vi "test4-EndNodeHandlesErrorForNotAllowedMessages.vi"(8 "error in (no error)":errorcluster, 11 "TestCase in":refnum<class "testcase-CSMChainMode.lvclass">) -> (0 "error out":errorcluster, 3 "TestCase out":refnum<class "testcase-CSMChainMode.lvclass">)   [LabVIEW 2017, in "testcase-CSMChainMode.lvclass"]
uses:
  testcase-CSMChainMode.lvclass
  src/user.lib/_NEVSTOP/Communicable State Machine(CSM)/_Support/Typedef/_CSM_MODE.ctl
  8deca385-1376-47bb-b92d-c44567c1a462.vi
  <vilib>/addons/_JKI Toolkits/VI Tester/TestCase.llb/TestCase.lvclass
  src/user.lib/_NEVSTOP/Communicable State Machine(CSM)/Communicable State Machine.lvlib
  C:/Program Files (x86)/National Instruments/LabVIEW 2017/vi.lib/addons/_JKI Toolkits/VI Tester/TestCase.llb/TestCase.lvclass
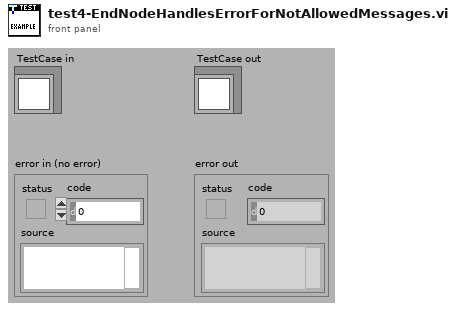
[diagram p1: front panel]
types:
  T1 = typedef "Communicable State Machine.lvlib/_CSM_MODE.ctl" = enum16{"Not Exist", "Stand Alone", "CSM", "Worker", "Worker Agent", "Chain Node", "Chain"}
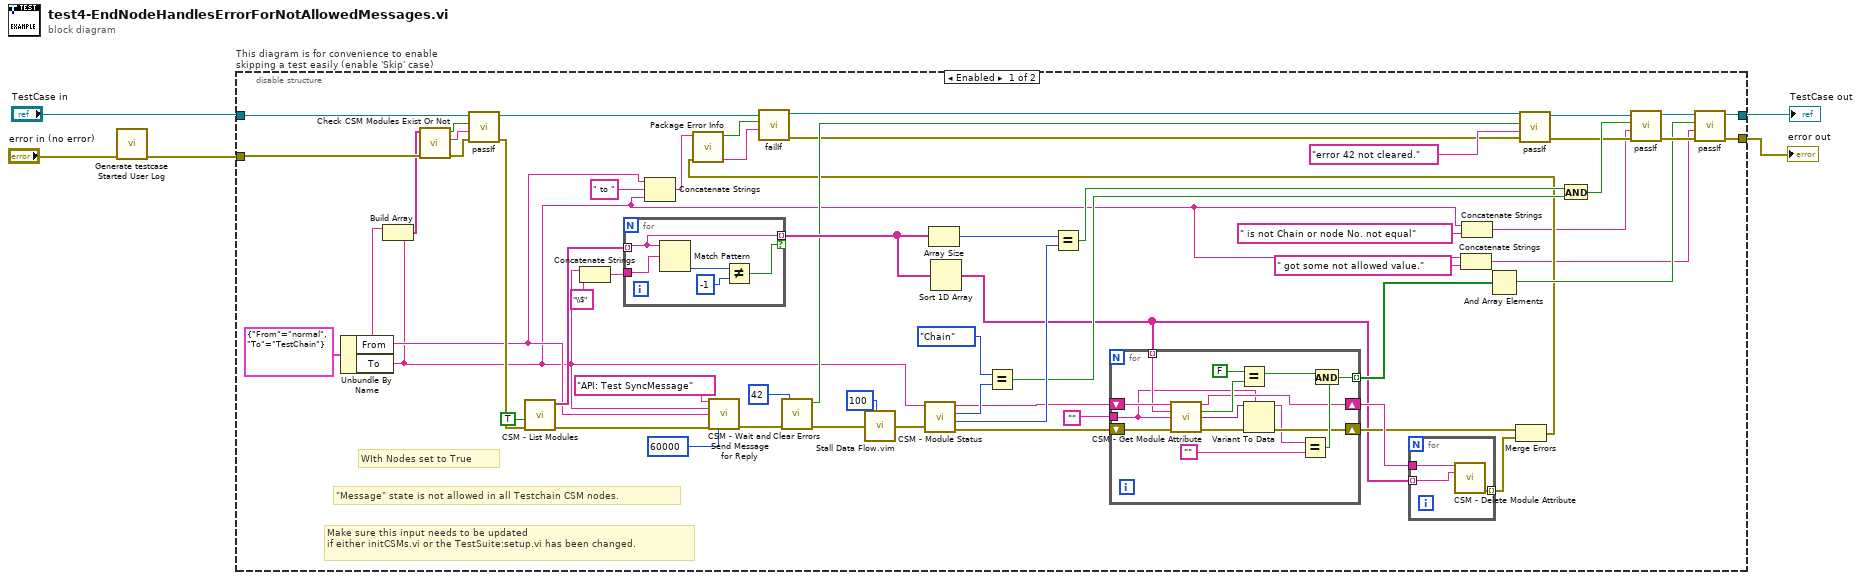
[diagram p0: block diagram]
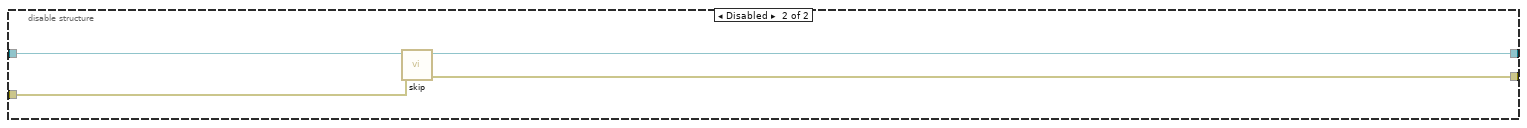
[diagram p2: hidden frame]
diagram:
  n1 = call "Generate testcase Started User Log.vi"("Error In"="error in (no error)") -> ("error out"=w1:errorcluster)  [unwired: 10 in]
  n2 = disable-structure "This diagram is for convenience to enable skipping a test easily (enable 'Skip' case)" shown="Enabled" {
    disable-tunnel: "TestCase in" -> [w20 w91]
    disable-tunnel: [w49 w89] -> w2
    disable-tunnel: [w48 w90] -> w4
    disable-tunnel: w1 -> [w18 w88]
    frame Enabled {
      # "\"Message\" state is not allowed in all Testchain CSM nodes."
      # "Make sure this input needs to be updated \nif either initCSMs.vi or the TestSuite:setup.vi has been changed."
      # "WIth Nodes set to True"
      n3 = Unbundle By Name(cluster{"From":string, "To":string} {"From"="normal", "To"="TestChain"} ("Cluster")) -> ("From"=w12:string, "To"=w9:string)
      n4 = Build Array(w12, w9) -> (w17:string[])
      n5 = call "Check CSM Modules Exist Or Not.vi"("error in"=w18, "CSM names in"=w17) -> ("error out"=w26:errorcluster, "Debug string"=w27:string, "All Modules Exist?"=w28:bool)  [unwired: 7 in]
      n6 = call-dynamic "passIf.vi"("error in (no error)"=w26, "message (\"\")"=w27, "pass"=w28, "TestCase in"=w20) -> ("error out"=w16:errorcluster, "TestCase out"=w21:refnum<class "testcase-CSMChainMode.lvclass">)  [unwired: 6 in]
      n7 = call "CSM - List Modules.vi"("Error In"=w16, "With Nodes? (F)"=TRUE) -> ("error out"=w57:errorcluster, "Module Names"=w60:string[])  [unwired: 8 in]
      n8 = Concatenate Strings(w9, "\\$" ("string")) -> (w46:string)
      n9 = for {
        tunnel: w60 -> [w85] mode=indexing
        tunnel: [w85] -> w43 mode=indexing if=w84
        tunnel: w46 -> [w83]
        n10 = Match Pattern(string=w85, regular expression=w83) -> (offset past match=w87:i32)  [unwired: 1 in, 3 out]
        n11 = Not Equal?(x=w87, y=-1) -> (x != y?=w84:bool)
      }
      n12 = Concatenate Strings(w12, " to " ("string"), w9) -> (w22:string)
      n13 = call "CSM - Wait and Send Message for Reply.vi"("State"="API: Test SyncMessage", "Arguments (\"\")"=w9, "Target Module"=w12, "Error In (No Error)"=w57, "Response Timeout (-2 Using Global Settings)"=60000) -> ("error out"=w37:errorcluster)  [unwired: 7 in, 3 out]
      n14 = call <vilib>:"Clear Errors.vi"("error in (no error)"=w37, "specific error code to clear (0: all)"=42) -> ("error out"=w40:errorcluster, "specific error cleared?"=w29:bool)  [unwired: 4 in]
      n15 = call "Stall Data Flow.vim"("value in"=w40, "milliseconds to wait"=u32 100) -> ("value out"=w62:errorcluster)  [unwired: 1 out]
      n16 = call "CSM - Module Status.vi"("Error In"=w62, "CSM Name"=w9) -> ("error out"=w39:errorcluster, "#Nodes"=w56:i32, "Mode"=w58:T1, "CSM Name (Dup)"=w38:string)  [unwired: 5 in, 1 out]
      n17 = Array Size(array=w43) -> (size(s)=w42:i32)
      n18 = Sort 1D Array(array=w43) -> (sorted array=w33:string[])
      n19 = Equal?(x=_CSM_MODE."Chain" ("Mode 2"), y=w58) -> (x = y?=w54:bool)
      n20 = Equal?(x=w42, y=w56) -> (x = y?=w55:bool)
      n21 = for {
        shift-right: [w72] -> w44
        shift-left: w38 -> [w78]
        shift-right: [w73] -> w34
        shift-left: w39 -> [w76]
        tunnel: "" -> [w69]
        tunnel: w33 -> [w77] mode=indexing
        tunnel: [w79] -> w41 mode=indexing
        n22 = call "CSM - Get Module Attribute.vi"("CSM Name"=w78, "Attribute"=w77, "Default Value (Empty Variant)"=w69, "Error In"=w76) -> ("CSM Name (Dup)"=w72:string, "Found"=w75:bool, "Value"=w71:variant, "error out"=w74:errorcluster)  [unwired: 7 in, 1 out]
        n23 = Equal?(x=FALSE, y=w75) -> (x = y?=w81:bool)
        n24 = Variant To Data(error in=w74, type=w69, Variant=w71) -> (data=w68:string, error out=w73:errorcluster)
        n25 = Equal?(x=w68, y="") -> (x = y?=w80:bool)
        n26 = And(x=w81, y=w80) -> (x .and. y?=w79:bool)
      }
      n27 = for {
        tunnel: [w67] -> w50 mode=indexing
        tunnel: w44 -> [w66]
        tunnel: w33 -> [w65] mode=indexing
        n28 = call "CSM - Delete Module Attribute.vi"("CSM Name"=w66, "Attribute"=w65) -> ("error out"=w67:errorcluster)  [unwired: 10 in, 3 out]
      }
      n29 = Concatenate Strings(w9, " got some not allowed value." ("string")) -> (w7:string)
      n30 = Concatenate Strings(w9, " is not Chain or node No. not equal" ("string")) -> (w11:string)
      n31 = And Array Elements(Boolean array=w41) -> (logical AND=w35:bool)
      n32 = Merge Errors(w34, w50) -> (w14:errorcluster)
      n33 = call "Package Error Info.vi"("error in"=w14, "String in"=w22) -> ("packed error info out"=w24:string, "error status"=w25:bool)  [unwired: 8 in]
      n34 = call-dynamic "failIf.vi"("message (\"\")"=w24, "fail"=w25, "TestCase in"=w21) -> ("error out"=w13:errorcluster, "TestCase out"=w19:refnum<class "testcase-CSMChainMode.lvclass">)  [unwired: 7 in]
      n35 = call-dynamic "passIf.vi"("error in (no error)"=w13, "message (\"\")"="error 42 not cleared." ("message (\"\")"), "pass"=w29, "TestCase in"=w19) -> ("error out"=w30:errorcluster, "TestCase out"=w31:refnum<class "testcase-CSMChainMode.lvclass">)  [unwired: 6 in]
      n36 = And(x=w55, y=w54) -> (x .and. y?=w53:bool)
      n37 = call-dynamic "passIf.vi"("error in (no error)"=w30, "message (\"\")"=w11, "pass"=w53, "TestCase in"=w31) -> ("error out"=w51:errorcluster, "TestCase out"=w52:refnum<class "testcase-CSMChainMode.lvclass">)  [unwired: 6 in]
      n38 = call-dynamic "passIf.vi"("error in (no error)"=w51, "message (\"\")"=w7, "pass"=w35, "TestCase in"=w52) -> ("error out"=w48:errorcluster, "TestCase out"=w49:refnum<class "testcase-CSMChainMode.lvclass">)  [unwired: 6 in]
    }
    frame Disabled {
      # "skip test result while test is under development"
      n39 = call <vilib>:"skip.vi"("error in (no error)"=w88, "TestCase in"=w91) -> ("error out"=w90:errorcluster, "TestCase out"=w89:refnum<class "testcase-CSMChainMode.lvclass">)  [unwired: 8 in]
    }
  }
  "error out" <- w4
  "TestCase out" <- w2
